vi "SOM Host.vi"() -> ()   [LabVIEW 2014]
uses:
  <vilib>/FPGAPlugInAG/sbRIO-9651/niLvFpga_Open_sbRIO-9651.vi
  <vilib>/rvi/interface/common/dynamic/niFpgaDynamicAddResources.vi
  <vilib>/FPGAPlugInAG/Dynamic/niLvFpga_Run_Dynamic.vi
  <vilib>/Utility/error.llb/Error Cluster From Error Code.vi
  <vilib>/rvi/errors/niLvFpgaAdjustHostInterfaceError.vi
  <vilib>/FPGAPlugInAG/Dynamic/niLvFpga_Close_Dynamic.vi
  <vilib>/rvi/interface/nirviOpenFPGA/nirviOpenFPGA.xnode
  FPGA Bitfiles/MAXREFDES5-4Chan_FPGATarget_SPIFPGA_gfIIDYSWaX0.lvbitx
  SPI FPGA.vi
  <vilib>/rvi/interface/nirviMethod/nirviMethod.xnode
  <vilib>/rvi/interface/nirviCloseFPGA/nirviCloseFPGA.xnode
  <vilib>/rvi/errors/niLvFpgaMergeErrorWithErrorCode.vi
  <vilib>/FPGAPlugInAG/Dynamic/niLvFpga_ReadFifo_Dynamic.vi
  <vilib>/FPGAPlugInAG/Dynamic/niLvFpga_StartFifo_Dynamic.vi
panel:
  out "RT Loop Iterations":i32
  out "Waveform Chart 2":u64[](graph)
  out "Waveform Chart":cluster{u64, u64, u64, u64}(graph)
  in  "stop":bool
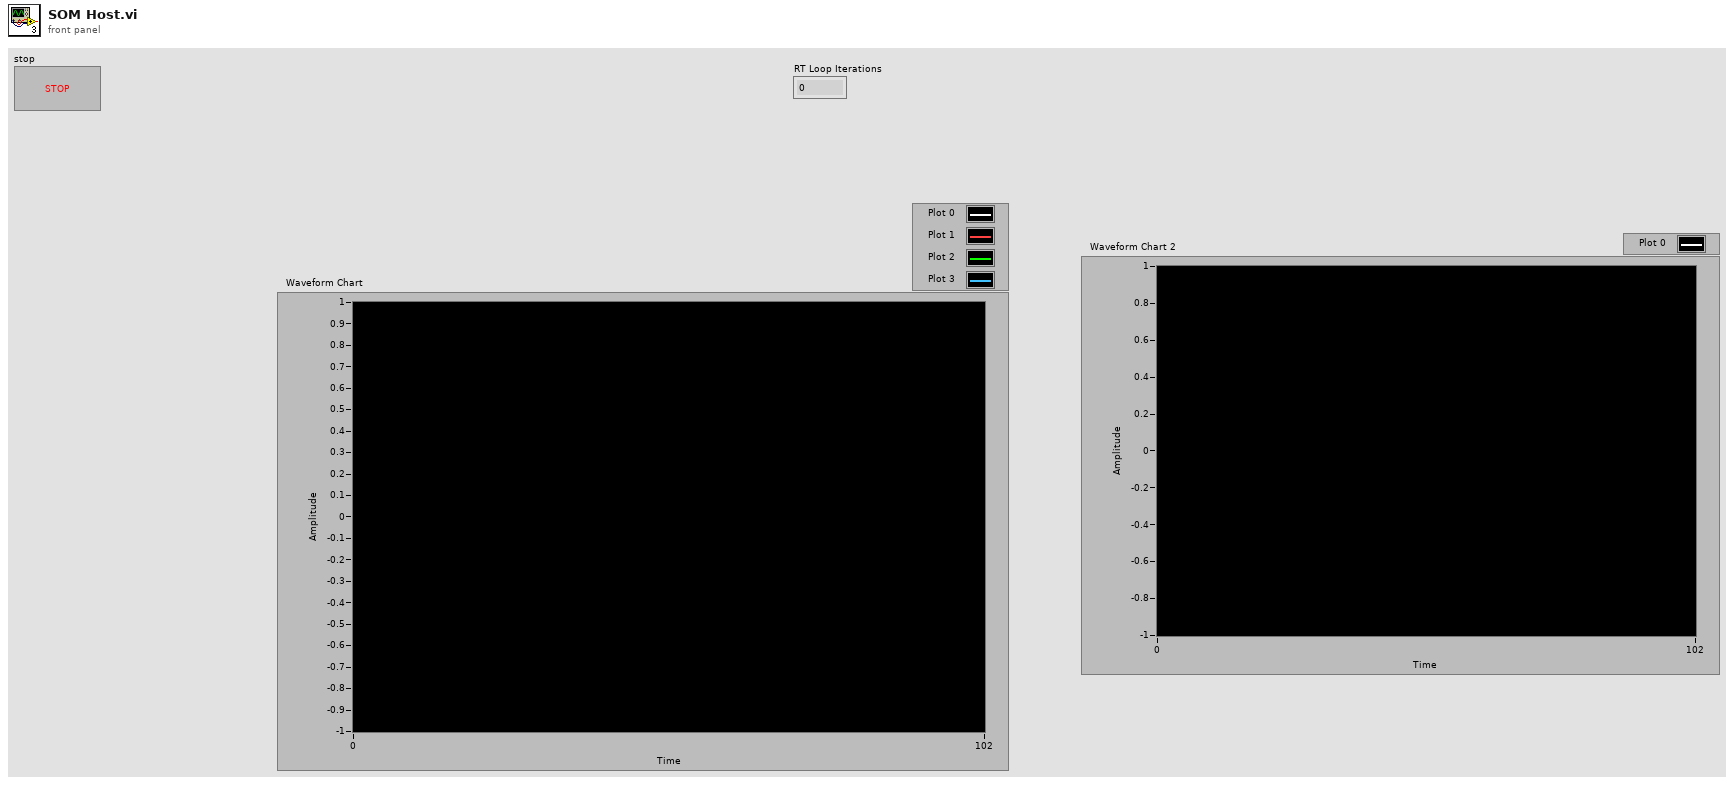
[diagram p1: front panel]
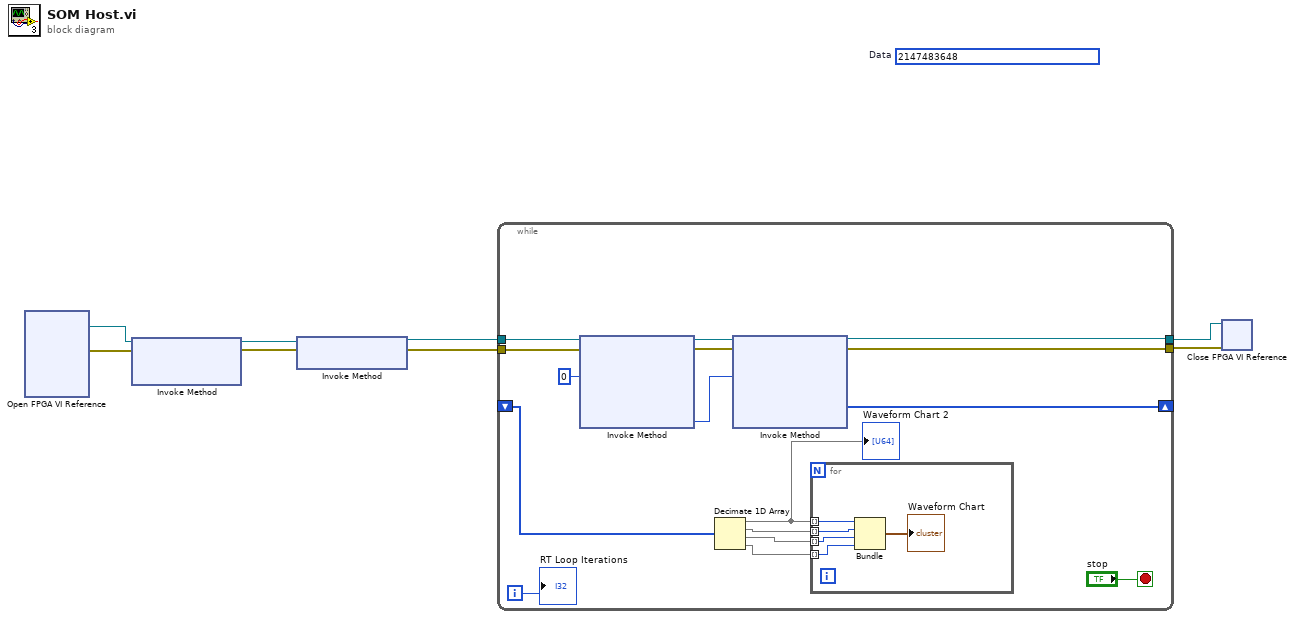
[diagram p0: block diagram]
diagram:
  (unwired) u64 2147483648  # Data
  n1 = xnode "Open FPGA VI Reference"() -> ("FPGA VI Reference Out"=w7:refnum<k20>, "error out"=w8:errorcluster)  [unwired: 2 in]
  n2 = xnode "Invoke Method"("FPGA VI Reference In"=w7, "error in"=w8) -> ("FPGA VI Reference Out"=w5:refnum<k20>, "error out"=w6:errorcluster)  [unwired: 1 in]
  n3 = xnode "Invoke Method"("FPGA VI Reference In"=w5, "error in"=w6) -> ("FPGA VI Reference Out"=w3:refnum<k20>, "error out"=w4:errorcluster)
  n4 = while {
    tunnel: w4 -> [w24]
    tunnel: w3 -> [w23]
    tunnel: [w10] -> w2
    tunnel: [w9] -> w1
    shift-right: [w17] -> _
    shift-left: _ -> [w16]
    i -> [w11]
    stop <- "stop" stop-if-true
    n5 = xnode "Invoke Method"("FPGA VI Reference In"=w23, "error in"=w24, "Number of Elements"=u32 0) -> ("FPGA VI Reference Out"=w21:refnum<k20>, "error out"=w20:errorcluster, "Elements Remaining"=w19:u32)  [unwired: 1 in, 1 out]
    n6 = Decimate 1D Array(w16) -> (w12:u64[], w15:u64[], w14:u64[], w13:u64[])
    "Waveform Chart 2" <- w12
    n7 = xnode "Invoke Method"("FPGA VI Reference In"=w21, "error in"=w20, "Number of Elements"=w19) -> ("FPGA VI Reference Out"=w9:refnum<k20>, "error out"=w10:errorcluster, "Data"=w17:u64[])  [unwired: 1 in, 1 out]
    n8 = for {
      tunnel: w12 -> [w29] mode=indexing
      tunnel: w15 -> [w28] mode=indexing
      tunnel: w14 -> [w27] mode=indexing
      tunnel: w13 -> [w26] mode=indexing
      n9 = Bundle(w29, w28, w27, w26) -> (→"Waveform Chart":cluster{u64, u64, u64, u64})  [unwired: 1 in]
    }
    "RT Loop Iterations" <- w11
  }
  n10 = xnode "Close FPGA VI Reference"("FPGA VI Reference In"=w1, "error in"=w2) -> ()  [unwired: 1 out]
